vi "Bridge Bias Close.vi"(8 "error in":errorcluster, 11 "bridge in":T1 {"TWM"."f-list [Hz]" format="%#_6p"}) -> (0 "error out":errorcluster, 3 "bridge out":T1 {"TWM"."f-list [Hz]" format="%#_6p"})   [LabVIEW 2013]
doc: "Close DC bias compensator session."
uses:
  Bridge Session.ctl
  Bridge Type.ctl
  drivers/TWM client/TWM Session.ctl
  drivers/TWM client/TWM parameters.ctl
  drivers/TWM client/Meas Proc QWTB Uncertainty Mode.ctl
  Bridge Bias Session.ctl
  Bridge Bias Type.ctl
  <vilib>/Utility/error.llb/Error Cluster From Error Code.vi
  <vilib>/ErrorRing/Error Ring.xnode
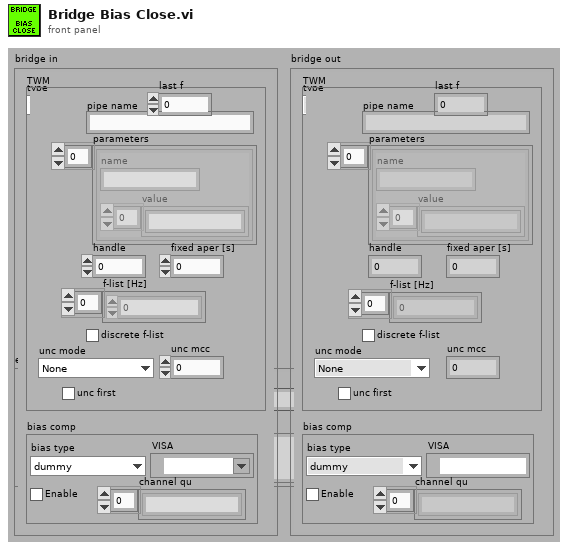
[diagram p1: front panel]
types:
  T1 = typedef "Bridge Session.ctl" = cluster{"type":T2, "TWM":T3, "last f":dbl, "bias comp":T6}
  T2 = typedef "Bridge Type.ctl" = enum16{"TWM client", "dummy"}
  T3 = typedef "TWM Session.ctl" = cluster{"pipe name":string, "parameters":T4[], "handle":i32, "fixed aper [s]":dbl, "f-list [Hz]":dbl[], "discrete f-list":bool, "unc mode":T5, "unc mcc":i32, "unc first":bool}
  T4 = typedef "TWM parameters.ctl" = cluster{"name":string, "value":string[]}
  T5 = typedef "Meas Proc QWTB Uncertainty Mode.ctl" = enum16{"None", "GUF", "Monte Carlo"}
  T6 = typedef "Bridge Bias Session.ctl" = cluster{"bias type":T7, "VISA":refnum<visa-resource-name>, "Enable":bool, "channel qu":string[]}
  T7 = typedef "Bridge Bias Type.ctl" = enum16{"dummy", "CMI LiBbias V1.0"}
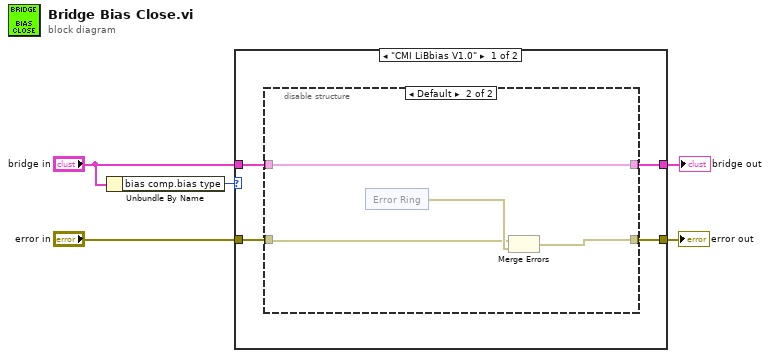
[diagram p0: block diagram]
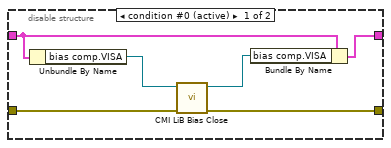
[diagram p2: hidden frame]
diagram:
  n1 = Unbundle By Name("bridge in") -> ("bias comp.bias type"=w5:T7)
  n2 = case shown="\"CMI LiBbias V1.0\"" w5 {
    tunnel: "error in" -> [w7 w26]
    tunnel: [w6 w26] -> w3
    tunnel: "bridge in" -> [w9 w25]
    tunnel: [w8 w25] -> w1
    frame "CMI LiBbias V1.0" {
      n3 = disable-structure shown="Default" {
        disable-tunnel: w9 -> [w15 w16]
        disable-tunnel: [w14 w16] -> w8
        disable-tunnel: w7 -> [w13 w18]
        disable-tunnel: [w12 w17] -> w6
        frame condition #0 (active) {
          n4 = Unbundle By Name(w15) -> ("bias comp.VISA"=w11:refnum<visa-resource-name>)
          n5 = call "CMI LiB Bias Close.vi"("error in"=w13, "VISA in"=w11) -> ("error out"=w12:errorcluster, "VISA out"=w10:refnum<visa-resource-name>)  [unwired: 8 in]
          n6 = Bundle By Name(cluster=w15, "bias comp.VISA"=w10) -> (w14:T1)
        }
        frame condition #1 {
          n7 = xnode "Error Ring"() -> ("error out"=w19:errorcluster)
          n8 = Merge Errors(w18, w19) -> (w17:errorcluster)
        }
      }
    }
    frame Default {
    }
  }
  "error out" <- w3
  "bridge out" <- w1
